vi "merge_two_exp.vi"(0 "all exp to average":refnum<class "Experiment.lvclass">[](array[class]), 3 "error in (no error)":errorcluster) -> (7 "averaged without bad points":dbl[][](array[numeric]), 8 "wavelength new":dbl[](array[numeric]), 9 "Array":cluster{"X pixels":dbl, "Y pixels":dbl}[](array[cluster]), 10 "sortie d'erreur":errorcluster)   [LabVIEW 2020, in "Experiment.lvclass"]
uses:
  Classes/Experiments/Experiment.lvclass
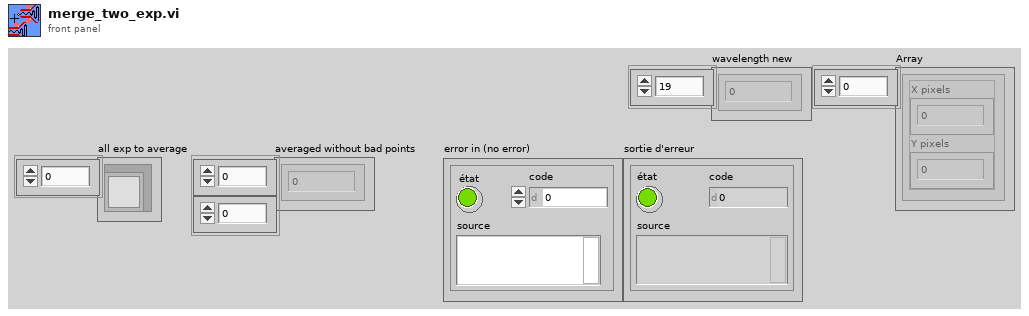
[diagram p1: front panel]
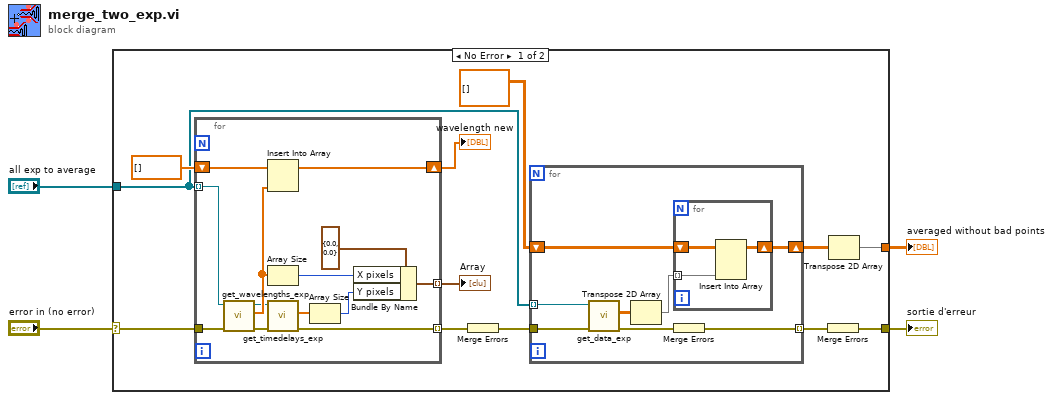
[diagram p0: block diagram]
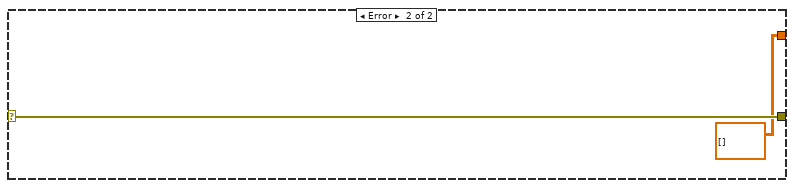
[diagram p2: hidden frame]
diagram:
  n1 = case shown="No Error" "error in (no error)" {
    selector: "error in (no error)" -> [w10 w42]
    tunnel: "all exp to average" -> [w14 _]
    tunnel: [w6 dbl[][] []] -> w3
    tunnel: [w12 w42] -> w2
    frame No Error {
      n2 = for {
        tunnel: w14 -> [w40] mode=indexing
        shift-right: [w37] -> w15
        shift-left: dbl[] [] ("timedelays") -> [w38]
        tunnel: w10 -> [w39]
        tunnel: [w30] -> w9 mode=indexing
        tunnel: [w33] -> w5 mode=indexing
        n3 = call "get_wavelengths_exp.vi"("error in (no error)"=w39, "Experiment.lvclass in"=w40) -> ("error out"=w31:errorcluster, "wavelengths"=w36:dbl[], "Experiment.lvclass out"=w32:refnum<class "Experiment.lvclass">)  [unwired: 7 in]
        n4 = Insert Into Array(array=w38, new element=w36) -> (w37:dbl[])  [unwired: 1 in]
        n5 = Array Size(array=w36) -> (size(s)=w35:i32)
        n6 = call "get_timedelays_exp.vi"("error in (no error)"=w31, "Experiment.lvclass in"=w32) -> ("error out"=w30:errorcluster, "timedelays"=w29:dbl[])  [unwired: 7 in, 1 out]
        n7 = Array Size(array=w29) -> (size(s)=w28:i32)
        n8 = Bundle By Name(cluster=cluster{"X pixels":dbl, "Y pixels":dbl} {"X pixels"=0.0, "Y pixels"=0.0} ("Size of exp"), "X pixels"=w35, "Y pixels"=w28) -> (w33:cluster{"X pixels":dbl, "Y pixels":dbl})
      }
      "wavelength new" <- w15
      "Array" <- w5
      n9 = Merge Errors(w9) -> (w11:errorcluster)
      n10 = for {
        tunnel: [w23] -> w13 mode=indexing
        tunnel: w11 -> [w22]
        tunnel: w14 -> [w21] mode=indexing
        shift-right: [w19] -> w7
        shift-left: sgl[][] [] ("Data") -> [w20]
        n11 = call "get_data_exp.vi"("error in (no error)"=w22, "Experiment.lvclass in"=w21) -> ("error out"=w24:errorcluster, "Data"=w18:sgl[][])  [unwired: 7 in, 1 out]
        n12 = Transpose 2D Array(2D array=w18) -> (transposed array=w17:sgl[][])
        n13 = for {
          shift-right: [w25] -> w19
          shift-left: w20 -> [w27]
          tunnel: w17 -> [w26] mode=indexing
          n14 = Insert Into Array(array=w27, new element=w26) -> (w25:sgl[][])  [unwired: 2 in]
        }
        n15 = Merge Errors(w24) -> (w23:errorcluster)
      }
      n16 = Merge Errors(w13) -> (w12:errorcluster)
      n17 = Transpose 2D Array(2D array=w7) -> (transposed array=w6:sgl[][])
    }
    frame Error {
    }
  }
  "averaged without bad points" <- w3
  "sortie d'erreur" <- w2
